vi "FPGA Threshold.vi"   [LabVIEW 2013, in "NI_EP_Protection_FPGA.lvlib"]
doc: "Detects the input energizing quantity <B>G</B> for deciding whether <B>G</B> turns to a pick-up signal according to <B>pick-up settings</B>."
uses:
  <vilib>/addons/Electrical Power/Protection/NI_EP_Protection_FPGA.lvlib
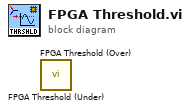
[diagram p0: block diagram]
diagram:
  n1 = call <vilib>:"FPGA Threshold (Under).vi"() -> ()  [unwired: 9 in, 3 out]
  n2 = call <vilib>:"FPGA Threshold (Over).vi"() -> ()  [unwired: 9 in, 3 out]
